vi "Get Listbox Row.vi"(8 "error in":errorcluster, 9 "Indicator?":bool, 10 "PWM Name":string, 11 "Node Ptr":T1 format="%.0x") -> (0 "error out":errorcluster, 3 "Listbox row":string[](array[string]))   [LabVIEW 2013, in "PWM System Explorer.lvlib"]
uses:
  PWM System Explorer.lvlib
  <vilib>/NI Veristand/Custom Device API/Custom Device Item Ref.ctl
  Shared/Constants.vi
  <vilib>/NI Veristand/Custom Device Tools/Custom Device Utility Library/NI VeriStand - Search for Item by Name.vi
  <vilib>/NI Veristand/Custom Device API/Get Item Property (Double).vi
  <vilib>/NI Veristand/Custom Device Tools/Custom Device Utility Library/Custom Device Utility Library.lvlib
  Shared/PWM Shared.lvlib
  <vilib>/NI Veristand/Custom Device API/Custom Device API.lvlib
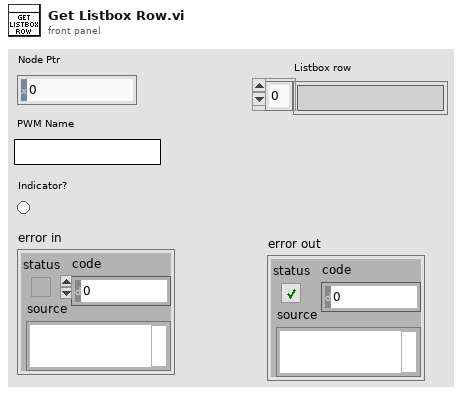
[diagram p1: front panel]
types:
  T1 = typedef "Custom Device API.lvlib/Custom Device Item Ref.ctl" = u64
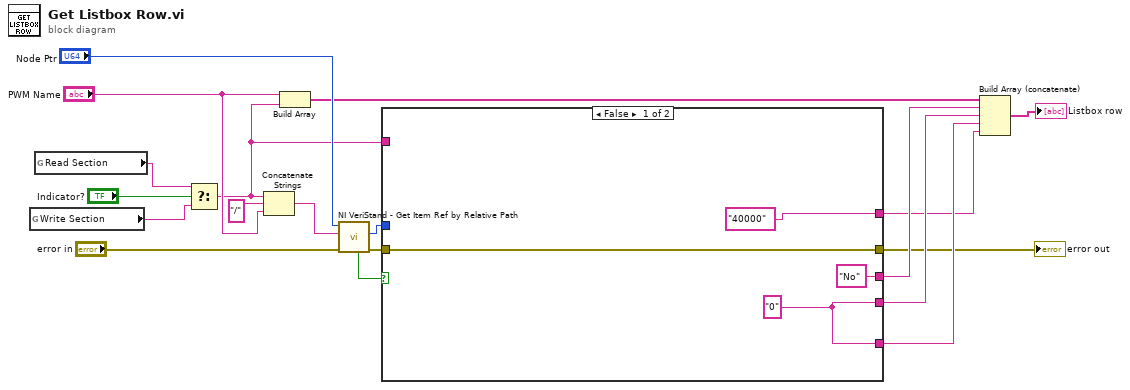
[diagram p0: block diagram]
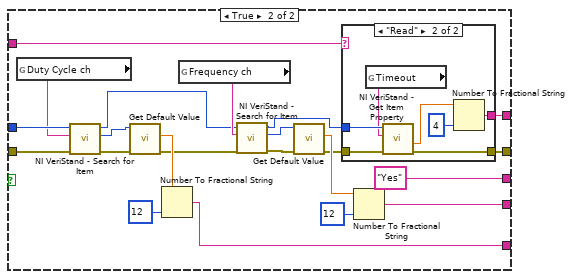
[diagram p2: hidden frame]
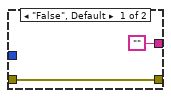
[diagram p3: hidden frame]
diagram:
  n1 = global read "Constants.vi" "Write Section"() -> (w18:string)
  n2 = global read "Constants.vi" "Read Section"() -> (w19:string)
  n3 = Select(t=w19, s="Indicator?", f=w18) -> (s? t:f=w1:string)
  n4 = Concatenate Strings(w1, "/" ("string"), "PWM Name") -> (w14:string)
  n5 = Build Array("PWM Name", w1) -> (w8:string[])
  n6 = call <vilib>:"NI VeriStand - Get Item Ref by Relative Path.vi"("error in"="error in", "Relative Item Path"=w14, "Section Ref in"="Node Ptr") -> ("error out"=w10:errorcluster, "Item Ref"=w12:T1, "Found"=w13:bool)  [unwired: 5 in, 1 out]
  n7 = case shown="False" w13 {
    tunnel: w12 -> [_ w45]
    tunnel: [w23 w29] -> w3
    tunnel: w10 -> [w23 w38]
    tunnel: [w21 w37] -> w5
    tunnel: [w21 w36] -> w6
    tunnel: ["No" ("string") "Yes" ("string")] -> w7
    tunnel: ["40000" w25] -> w2
    tunnel: w1 -> [_ w24]
    frame False {
      w21 = "0"
    }
    frame True {
      n8 = global read "Constants.vi" "Duty Cycle ch"() -> (w43:string)
      n9 = call-poly <vilib>:"NI VeriStand - Search for Item.vi"("error in"=w38, "Item Name"=w43, "Section Ref in"=w45) -> ("error out"=w44:errorcluster, "Item Ref"=w42:T1, "Section Ref out"=w27:T1)  [unwired: 5 in, 1 out]
      n10 = call "Get Default Value.vi"("error in (no error)"=w44, "Item Ref in"=w42) -> ("error out"=w32:errorcluster, "DefaultValue"=w40:dbl)  [unwired: 7 in, 1 out]
      n11 = Number To Fractional String(number=w40, precision (6)=i16 12) -> (F-format string=w37:string)  [unwired: 2 in]
      n12 = global read "Constants.vi" "Frequency ch"() -> (w31:string)
      n13 = call-poly <vilib>:"NI VeriStand - Search for Item.vi"("error in"=w32, "Item Name"=w31, "Section Ref in"=w27) -> ("error out"=w33:errorcluster, "Item Ref"=w28:T1, "Section Ref out"=w26:T1)  [unwired: 5 in, 1 out]
      n14 = call "Get Default Value.vi"("error in (no error)"=w33, "Item Ref in"=w28) -> ("error out"=w30:errorcluster, "DefaultValue"=w34:dbl)  [unwired: 7 in, 1 out]
      n15 = case shown="\"Read\"" w24 {
        tunnel: w30 -> [w47 w54]
        tunnel: [w47 w53] -> w29
        tunnel: w26 -> [_ w52]
        tunnel: ["" w50] -> w25
        frame "False", Default {
        }
        frame "Read" {
          n16 = global read "Constants.vi" "Timeout"() -> (w48:string)
          n17 = call-poly <vilib>:"NI VeriStand - Get Item Property.vi"("error in (no error)"=w54, "Property Name"=w48, "Item Ref in"=w52) -> ("error out"=w53:errorcluster, "Value"=w49:dbl)  [unwired: 5 in, 2 out]
          n18 = Number To Fractional String(number=w49, precision (6)=i16 4) -> (F-format string=w50:string)  [unwired: 2 in]
        }
      }
      n19 = Number To Fractional String(number=w34, precision (6)=i16 12) -> (F-format string=w36:string)  [unwired: 2 in]
    }
  }
  "error out" <- w3
  n20 = Build Array (concatenate)(w8, w7, w6, w5, w2) -> (→"Listbox row":string[])
